vi "SLSC Update Channels State to Tree Control.vi"(0 "Property tree":refnum<vi>, 1 "Update Only?":bool, 5 "SLSC Output Tree":T3(array[cluster]), 7 "Channels to \"enable\"":string[](array[string]), 9 "Channel Values":dbl[](array[numeric]), 11 "error in (no error)":errorcluster, 13 "string enums":T2(array[cluster])) -> (15 "error out":errorcluster)   [LabVIEW 2017, in "SLSC Tree Control.lvlib"]
doc: "Updates the tree control with the new information from the SLSC Output Tree. It also changes the icons according to to the state of the channel."
uses:
  SLSC Tree Control.lvlib
  Ctrl/EnumValue.ctl
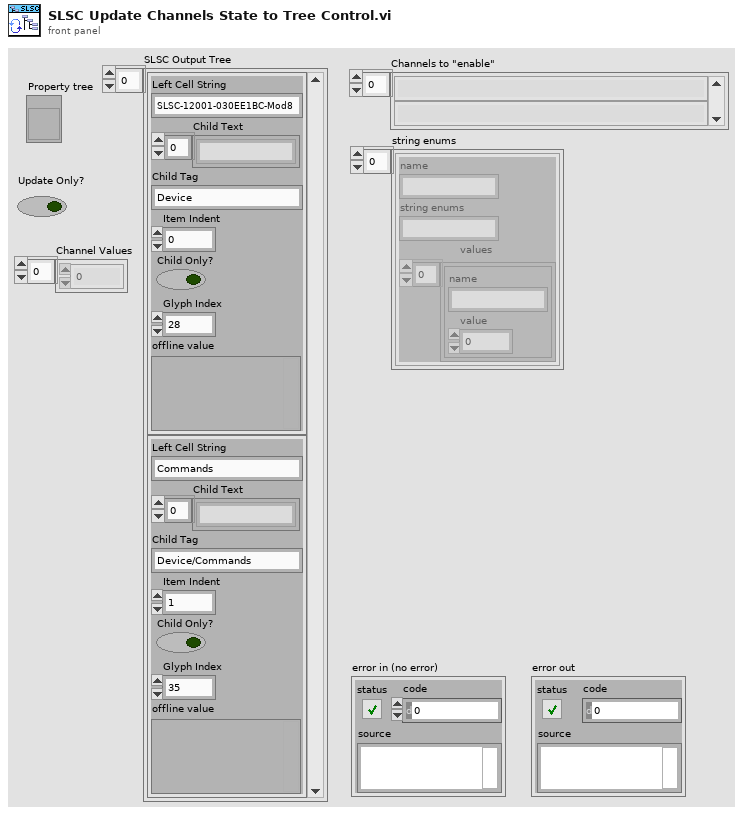
[diagram p1: front panel]
types:
  T1 = typedef "EnumValue.ctl" = cluster{"name":string, "value":i32}
  T2 = cluster{"name":string, "string enums":string, "values":T1[]}[]
  T3 = cluster{"Left Cell String":string, "Child Text":string[], "Child Tag":string, "Item Indent":i32, "Child Only?":bool, "Glyph Index":i32, "offline value":variant}[]
  T4 = cluster{"Left Cell String":string, "Child Text":string[], "Child Tag":string, "Item Indent":i32, "Child Only?":bool, "Glyph Index":i32}
  T5 = cluster{"Left Cell String":string, "Child Text":string[], "Child Tag":string, "Item Indent":i32, "Child Only?":bool, "Glyph Index":i32}[]
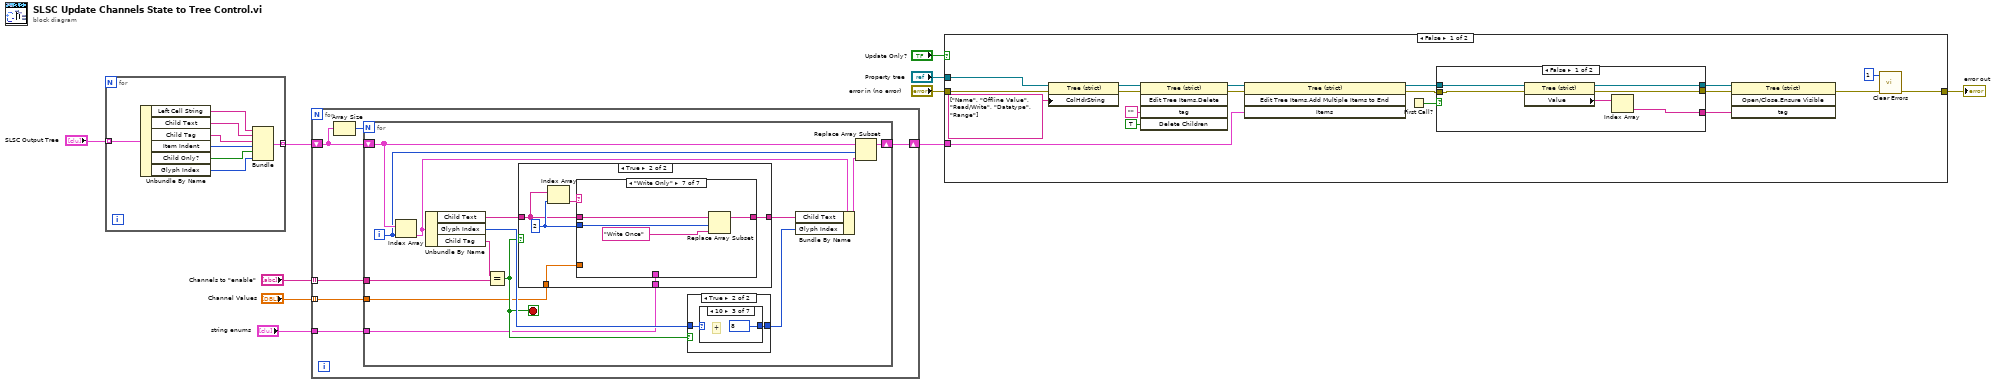
[diagram p0: block diagram]
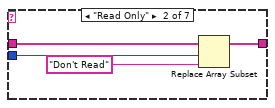
[diagram p4: hidden frame]
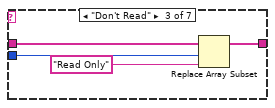
[diagram p5: hidden frame]
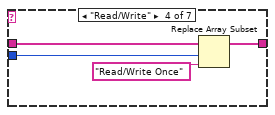
[diagram p6: hidden frame]
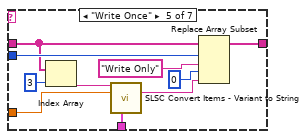
[diagram p7: hidden frame]
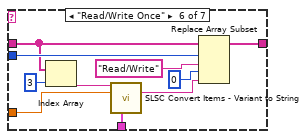
[diagram p8: hidden frame]
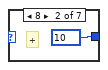
[diagram p11: hidden frame]
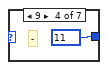
[diagram p12: hidden frame]
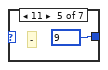
[diagram p13: hidden frame]
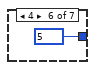
[diagram p14: hidden frame]
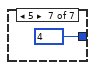
[diagram p15: hidden frame]
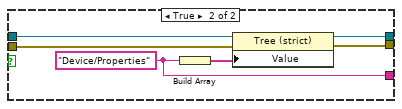
[diagram p16: hidden frame]
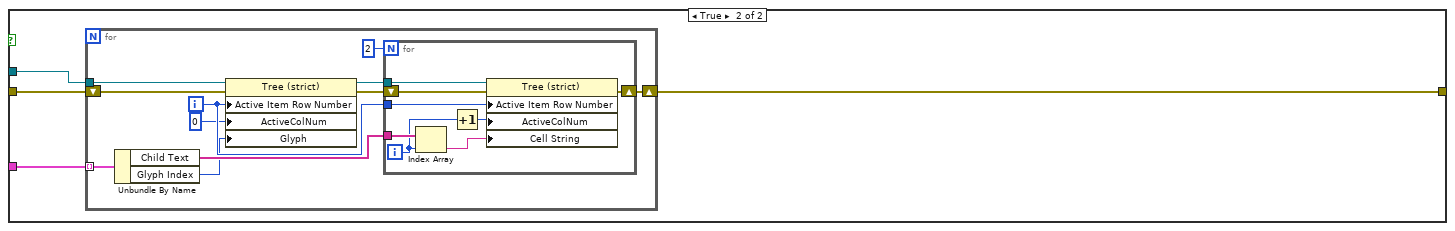
[diagram p17: hidden frame]
diagram:
  n1 = for {
    tunnel: "SLSC Output Tree" -> [w18] mode=indexing
    tunnel: [w11] -> w2 mode=indexing
    n2 = Unbundle By Name(w18) -> ("Left Cell String"=w17:string, "Child Text"=w16:string[], "Child Tag"=w15:string, "Item Indent"=w14:i32, "Child Only?"=w13:bool, "Glyph Index"=w12:i32)
    n3 = Bundle("Left Cell String"=w17, "Child Text"=w16, "Child Tag"=w15, "Item Indent"=w14, "Child Only?"=w13, "Glyph Index"=w12) -> (w11:T4)  [unwired: 1 in]
  }
  n4 = for {
    tunnel: "Channels to \"enable\"" -> [w21] mode=indexing
    shift-right: [w24] -> w8
    shift-left: w2 -> [w22]
    tunnel: "Channel Values" -> [w20] mode=indexing
    tunnel: "string enums" -> [w19]
    n5 = Array Size(array=w22) -> (size(s)=w23:i32)
    n6 = for {
      N: w23 -> [_]
      shift-right: [w37] -> w24
      shift-left: w22 -> [w38]
      tunnel: w21 -> [w33]
      tunnel: w20 -> [w26]
      tunnel: w19 -> [w25]
      i -> [w36]
      stop <- w29 stop-if-true
      n7 = Index Array(array=w38, index=w36) -> (element=w32:T4)
      n8 = Unbundle By Name(w32) -> ("Child Text"=w27:string[], "Glyph Index"=w30:i32, "Child Tag"=w34:string)
      n9 = Equal?(x=w34, y=w33) -> (x = y?=w29:bool)
      n10 = case shown="True" w29 {
        tunnel: [w39 w45] -> w28
        tunnel: w27 -> [w39 w43]
        tunnel: w26 -> [_ w41]
        tunnel: w25 -> [_ w40]
        frame False {
        }
        frame True {
          w44 = 2 ("index")
          n11 = Index Array(array=w43, index=w44) -> (element=w42:string)
          n12 = case shown="\"Write Only\"" w42 {
            tunnel: w43 -> [w46 w50 w54 w58 w65 w75 w82]
            tunnel: [w46 w49 w53 w57 w68 w78 w81] -> w45
            tunnel: w44 -> [_ w48 w52 w56 w67 w77 w80]
            tunnel: w41 -> [_ _ _ _ w62 w72 _]
            tunnel: w40 -> [_ _ _ _ w61 w71 _]
            frame Default {
            }
            frame "Read Only" {
              n13 = Replace Array Subset(array=w50, new element="Don't Read" ("new element/subarray"), index=w48) -> (w49:string[])
            }
            frame "Don't Read" {
              n14 = Replace Array Subset(array=w54, new element="Read Only" ("new element/subarray"), index=w52) -> (w53:string[])
            }
            frame "Read/Write" {
              n15 = Replace Array Subset(array=w58, new element="Read/Write Once" ("new element/subarray"), index=w56) -> (w57:string[])
            }
            frame "Write Once" {
              n16 = Index Array(array=w65, index=3) -> (element=w63:string)
              n17 = call "SLSC Convert Items - Variant to String.vi"("dataType"=w63, "value"=w62, "string enums"=w61) -> ("string offline data value"=w60:string)  [unwired: 8 in, 4 out]
              n18 = Replace Array Subset(array=w65, new element #1="Write Only" ("new element/subarray"), index #1=w67, new element #2=w60, index #2=0 ("index")) -> (w68:string[])
            }
            frame "Read/Write Once" {
              n19 = Index Array(array=w75, index=3) -> (element=w73:string)
              n20 = call "SLSC Convert Items - Variant to String.vi"("dataType"=w73, "value"=w72, "string enums"=w71) -> ("string offline data value"=w70:string)  [unwired: 8 in, 4 out]
              n21 = Replace Array Subset(array=w75, new element #1="Read/Write" ("new element/subarray"), index #1=w77, new element #2=w70, index #2=0 ("index")) -> (w78:string[])
            }
            frame "Write Only" {
              n22 = Replace Array Subset(array=w82, new element="Write Once" ("new element/subarray"), index=w80) -> (w81:string[])
            }
          }
        }
      }
      n23 = case shown="True" w29 {
        tunnel: [w83 w84] -> w31
        tunnel: w30 -> [w83 w85]
        frame False {
        }
        frame True {
          n24 = case shown="10" w85 {
            selector: w85 -> [w86 _ _ _ _ _ _]
            tunnel: [w86 10 8 11 9 5 4] -> w84
            frame Default {
            }
            frame 8 {
              # "+"
            }
            frame 10 {
              # "+"
            }
            frame 9 {
              # "-"
            }
            frame 11 {
              # "-"
            }
            frame 4 {
            }
            frame 5 {
            }
          }
        }
      }
      n25 = Bundle By Name(cluster=w32, "Child Text"=w28, "Glyph Index"=w31) -> (w35:T4)
      n26 = Replace Array Subset(array=w38, new element=w35, index=w36) -> (w37:T5)
    }
  }
  n27 = case shown="False" "Update Only?" {
    tunnel: "error in (no error)" -> [w106 w125]
    tunnel: [w94 w124] -> w1
    tunnel: "Property tree" -> [w105 w126]
    tunnel: w8 -> [w104 w127]
    frame False {
      n28 = property on="Property Node" class="Tree (strict)"(reference=w105, error in=w106, "ColHdrString"=string[] ["Name", "Offline Value", "Read/Write", "Datatype", "Range"]) -> (reference out=w103:refnum<vi>, error out=w108:errorcluster)
      n29 = invoke on="Invoke Node" class="Tree (strict)" method="Edit Tree Items.Delete"(reference=w103, error in=w108, "tag"="", "Delete Children"=TRUE ("Delete Children?")) -> (reference out=w102:refnum<vi>, error out=w107:errorcluster)  [unwired: 1 in, 3 out]
      n30 = invoke on="Invoke Node" class="Tree (strict)" method="Edit Tree Items.Add Multiple Items to End"(reference=w102, error in=w107, "Items"=w104) -> (reference out=w99:refnum<vi>, error out=w96:errorcluster)  [unwired: 1 in, 2 out]
      n31 = First Call?() -> (First Call?: T/F=w100:bool)
      n32 = case shown="False" w100 {
        tunnel: w99 -> [w115 w122]
        tunnel: [w116 w121] -> w98
        tunnel: [w114 w120] -> w97
        tunnel: w96 -> [w113 w119]
        tunnel: [w112 w118] -> w95
        frame False {
          n33 = property class="Tree (strict)"(reference=w115, error in=w113) -> (reference out=w116:refnum<vi>, error out=w112:errorcluster, "Value"=w117:string[])
          n34 = Index Array(array=w117) -> (element=w114:string)  [unwired: 1 in]
        }
        frame True {
          w120 = "Device/Properties" ("string")
          n35 = Build Array(w120) -> (w123:string[])
          n36 = property class="Tree (strict)"(reference=w122, error in=w119, "Value"=w123) -> (reference out=w121:refnum<vi>, error out=w118:errorcluster)
        }
      }
      n37 = invoke class="Tree (strict)" method="Open/Close.Ensure Visible"(reference=w98, error in=w95, "tag"=w97) -> (error out=w101:errorcluster)  [unwired: 1 in, 3 out]
      n38 = call <vilib>:"Clear Errors.vi"("error in (no error)"=w101, "specific error code to clear (0: all)"=1) -> ("error out"=w94:errorcluster)  [unwired: 4 in, 1 out]
    }
    frame True {
      n39 = for {
        tunnel: w127 -> [w137] mode=indexing
        tunnel: w126 -> [w135]
        shift-right: [w138] -> w124
        shift-left: w125 -> [w132]
        i -> [w131]
        n40 = Unbundle By Name(w137) -> ("Child Text"=w136:string[], "Glyph Index"=w129:i32)
        n41 = property class="Tree (strict)"(reference=w135, error in=w132, "Active Item Row Number"=w131, "ActiveColNum"=0 ("Active Cell:Active Column Number"), "Glyph"=w129) -> (reference out=w134:refnum<vi>, error out=w133:errorcluster)
        n42 = for {
          N: 2 -> [_]
          tunnel: w134 -> [w146]
          shift-right: [w144] -> w138
          shift-left: w133 -> [w145]
          tunnel: w131 -> [w142]
          tunnel: w136 -> [w143]
          i -> [w139]
          n43 = Index Array(array=w143, index=w139) -> (element=w140:string)
          n44 = Increment(x=w139) -> (x+1=w141:i32)
          n45 = property class="Tree (strict)"(reference=w146, error in=w145, "Active Item Row Number"=w142, "ActiveColNum"=w141, "Cell String"=w140) -> (error out=w144:errorcluster)  [unwired: 1 out]
        }
      }
    }
  }
  "error out" <- w1
